vi "_DRIVER_SHARED_INI_File-Handler.vi"(6 "INI-FileMethod":T2, 7 "section IN":string, 8 "error in (no error)":errorcluster, 9 "Value to write":string, 10 "key IN":string, 11 "Path File":string) -> (0 "error out":errorcluster, 2 "value Read":string, 3 "refnum out":T1)   [LabVIEW 2020]
doc: "File INI Handler, low level. Create, manage and close \"_HW_Configuration.ini\""
uses:
  TYPEDEF/_DRIVER_SHARED_TYPEDEF_INI-Method.ctl
  <vilib>/Utility/config.llb/Config Data RefNum.ctl
  <vilib>/Utility/config.llb/Read Key (String).vi
  <vilib>/Utility/config.llb/Write Key (String).vi
  <vilib>/Utility/config.llb/NI_LVConfig.lvlib
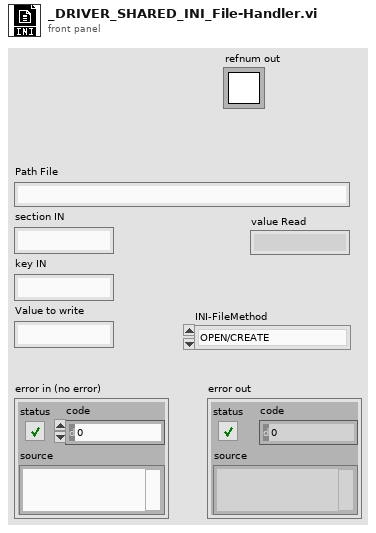
[diagram p1: front panel]
types:
  T1 = typedef "NI_LVConfig.lvlib/Config Data RefNum.ctl" = refnum<k1>
  T2 = typedef "_DRIVER_SHARED_TYPEDEF_INI-Method.ctl" = enum16{"OPEN/CREATE", "READ", "WRITE", "CLOSE", "NO_OP"}
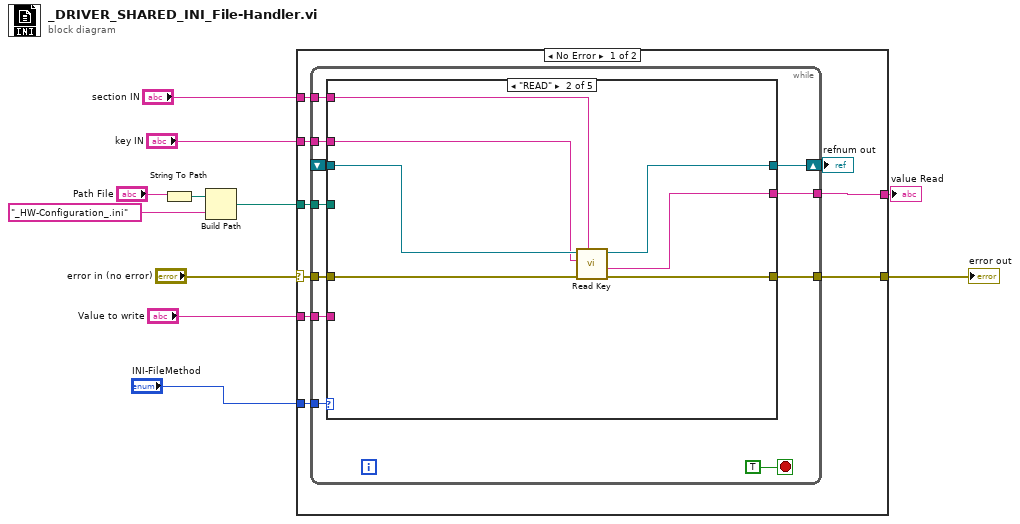
[diagram p0: block diagram]
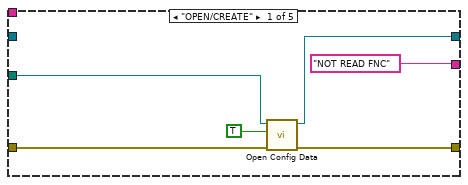
[diagram p2: hidden frame]
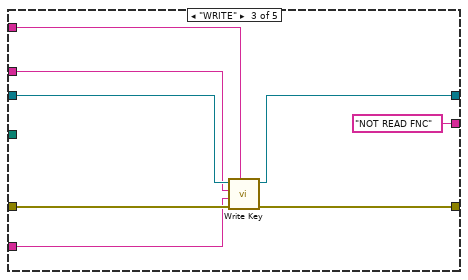
[diagram p3: hidden frame]
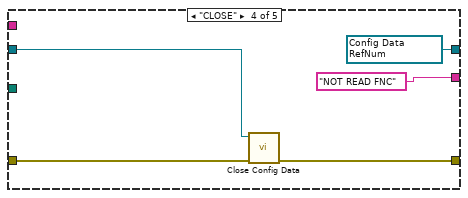
[diagram p4: hidden frame]
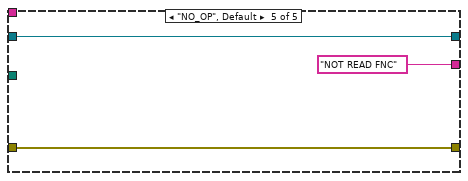
[diagram p5: hidden frame]
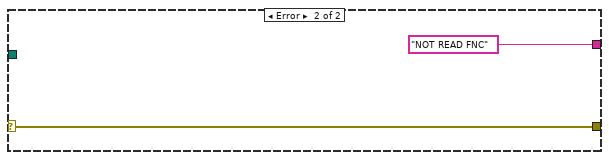
[diagram p6: hidden frame]
diagram:
  n1 = String To Path(string="Path File") -> (path=w9:path)
  n2 = Build Path(base path=w9, name or relative path="_HW-Configuration_.ini" ("Path File 2")) -> (appended path=w7:path)
  n3 = case shown="No Error" "error in (no error)" {
    selector: "error in (no error)" -> [w18 w61]
    tunnel: "INI-FileMethod" -> [w20 _]
    tunnel: w7 -> [w19 _]
    tunnel: [w17 w61] -> w5
    tunnel: "section IN" -> [w16 _]
    tunnel: "key IN" -> [w15 _]
    tunnel: [w14 "NOT READ FNC" ("value")] -> w2
    tunnel: "Value to write" -> [w13 _]
    frame No Error {
      n4 = while {
        tunnel: w20 -> [w30]
        tunnel: w19 -> [w29]
        shift-right: [w28] -> w12
        shift-left: _ -> [w27]
        tunnel: w18 -> [w26]
        tunnel: [w25] -> w17
        tunnel: w16 -> [w24]
        tunnel: w15 -> [w23]
        tunnel: [w22] -> w14
        tunnel: w13 -> [w21]
        stop <- TRUE stop-if-true
        n5 = case shown="\"READ\"" w30 {
          tunnel: w29 -> [w33 _ _ _ _]
          tunnel: [w36 w41 w49 w54 w60] -> w28
          tunnel: w27 -> [_ w42 w50 w55 w60]
          tunnel: w26 -> [w32 w44 w52 w57 w58]
          tunnel: [w35 w43 w51 w56 w58] -> w25
          tunnel: w24 -> [_ w40 w48 _ _]
          tunnel: w23 -> [_ w39 w47 _ _]
          tunnel: ["NOT READ FNC" ("value") w38 "NOT READ FNC" ("value") "NOT READ FNC" ("value") "NOT READ FNC" ("value")] -> w22
          tunnel: w21 -> [_ _ w46 _ _]
          frame "OPEN/CREATE" {
            n6 = call <vilib>:"Open Config Data.vi"("error in (no error)"=w32, "create file if necessary (T)"=TRUE, "configuration file path"=w33) -> ("error out"=w35:errorcluster, "refnum"=w36:T1)  [unwired: 6 in, 1 out]
          }
          frame "READ" {
            n7 = call-poly <vilib>:"Read Key.vi"("section"=w40, "error in (no error)"=w44, "key"=w39, "refnum"=w42) -> ("error out"=w43:errorcluster, "value"=w38:string, "refnum out"=w41:T1)  [unwired: 4 in, 1 out]
          }
          frame "WRITE" {
            n8 = call-poly <vilib>:"Write Key.vi"("section"=w48, "error in (no error)"=w52, "value"=w46, "key"=w47, "refnum"=w50) -> ("error out"=w51:errorcluster, "refnum out"=w49:T1)  [unwired: 4 in, 1 out]
          }
          frame "CLOSE" {
            w54 = T1 refnum items=["config data"] ("refnum out")
            n9 = call <vilib>:"Close Config Data.vi"("error in (no error)"=w57, "refnum"=w55) -> ("error out"=w56:errorcluster)  [unwired: 8 in, 1 out]
          }
          frame "NO_OP", Default {
          }
        }
      }
      "refnum out" <- w12
    }
    frame Error {
    }
  }
  "error out" <- w5
  "value Read" <- w2
